vi "Convert dBSPL to Pa.vi"(10 "dB SPL":dbl) -> (1 "Pa pk":dbl, 2 "Pa rms":dbl)   [LabVIEW 2022 SP3]
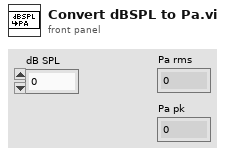
[diagram p1: front panel]
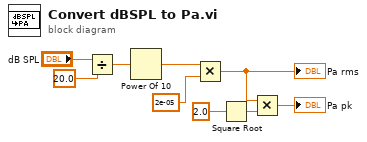
[diagram p0: block diagram]
diagram:
  n1 = Divide(x="dB SPL", y=20.0) -> (x/y=w7:dbl)
  n2 = Power Of 10(x=w7) -> (10^x=w6:dbl)
  n3 = Multiply(x=w6, y=2e-05) -> (x*y=w4:dbl)
  "Pa rms" <- w4
  n4 = Square Root(x=2.0) -> (sqrt(x)=w3:dbl)
  n5 = Multiply(x=w4, y=w3) -> (x*y=→"Pa pk":dbl)
